vi "Disconnect.vi"(8 "error in (no error)":errorcluster, 11 "Optris PI in":refnum<class "Optris PI.lvclass">) -> (0 "error out":errorcluster, 3 "Optris PI out":refnum<class "Optris PI.lvclass">)   [LabVIEW 2018, in "Optris PI.lvlib" / "Optris PI.lvclass"]
uses:
  Optris PI.lvclass
  <instrlib>/Optris PI/libirimager_direct_binding.lvlib
  PPLs/Thermal Camera/Parent/Thermal Camera.lvlibp/Thermal Camera.lvclass
  C:/AME Test Engineering/LabVIEW/PPLs/Thermal Camera/Parent/Thermal Camera.lvlibp/Thermal Camera.lvclass
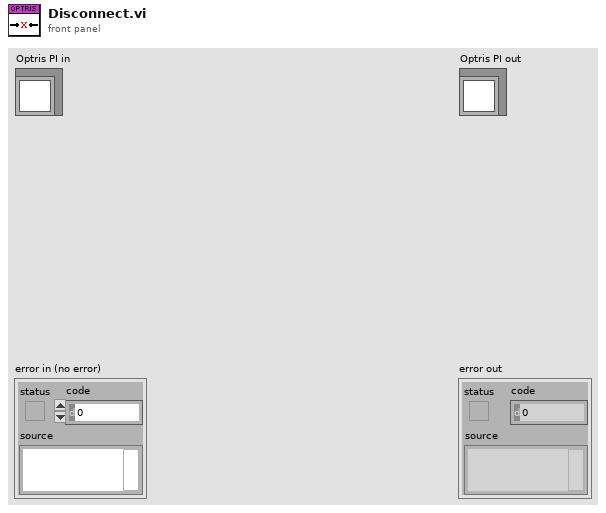
[diagram p1: front panel]
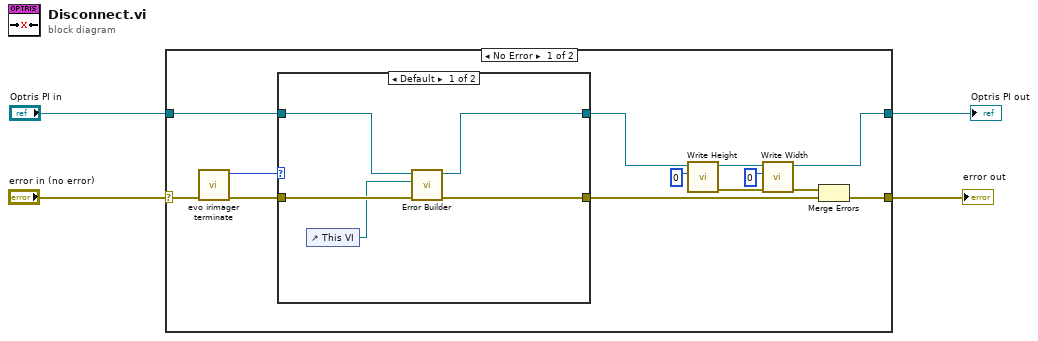
[diagram p0: block diagram]
diagram:
  n1 = case shown="No Error" "error in (no error)" {
    selector: "error in (no error)" -> [w17 w25]
    tunnel: "Optris PI in" -> [w9 w26]
    tunnel: [w16 w26] -> w2
    tunnel: [w5 w25] -> w1
    frame No Error {
      n2 = call <instrlib>:"evo irimager terminate.vi"("error in (no error)"=w17) -> ("error out"=w10:errorcluster, "function return"=w11:i32)  [unwired: 9 in]
      n3 = case shown="Default" w11 {
        tunnel: w10 -> [w22 w24]
        tunnel: [w19 w24] -> w6
        tunnel: w9 -> [w21 w23]
        tunnel: [w20 w23] -> w8
        frame Default {
          n4 = control-ref of="This VI"() -> (w18:refnum<vi>)
          n5 = call "Error Builder.vi"("error in (no error)"=w22, "This VI"=w18, "Optris PI in"=w21) -> ("Error out"=w19:errorcluster, "Optris PI out"=w20:refnum<class "Optris PI.lvclass">)  [unwired: 7 in]
        }
        frame 0 {
        }
      }
      n6 = call "Write Height.vi"("Height"=u32 0, "Thermal Camera in"=w8) -> ("error out"=w15:errorcluster, "Thermal Camera out"=w14:refnum<class "Optris PI.lvclass">)  [unwired: 8 in]
      n7 = call "Write Width.vi"("error in (no error)"=w15, "Width"=u32 0, "Thermal Camera in"=w14) -> ("error out"=w7:errorcluster, "Thermal Camera out"=w16:refnum<class "Optris PI.lvclass">)  [unwired: 7 in]
      n8 = Merge Errors(w7, w6) -> (w5:errorcluster)
    }
    frame Error {
    }
  }
  "error out" <- w1
  "Optris PI out" <- w2
